vi "Legal Position Check.vi"(7 "Parameters for Legal Movements":T1, 8 "error in (no error)":errorcluster, 10 "Scope Position":refnum<vi>, 11 "Tip Coordinates":refnum<vi>) -> (0 "error out":errorcluster, 2 "Crash":bool)   [LabVIEW 2012, in "Sciscan Scope Daemon.lvlib"]
uses:
  Sciscan Scope Daemon.lvlib
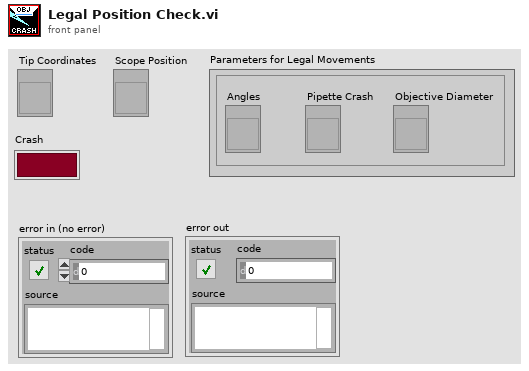
[diagram p1: front panel]
types:
  T1 = cluster{"Angles":refnum<vi>, "Objective Diameter":refnum<vi>, "Pipette Crash":refnum<vi>}
  T2 = cluster{"X [um]":dbl, "Y [um]":dbl, "Z [um]":dbl}
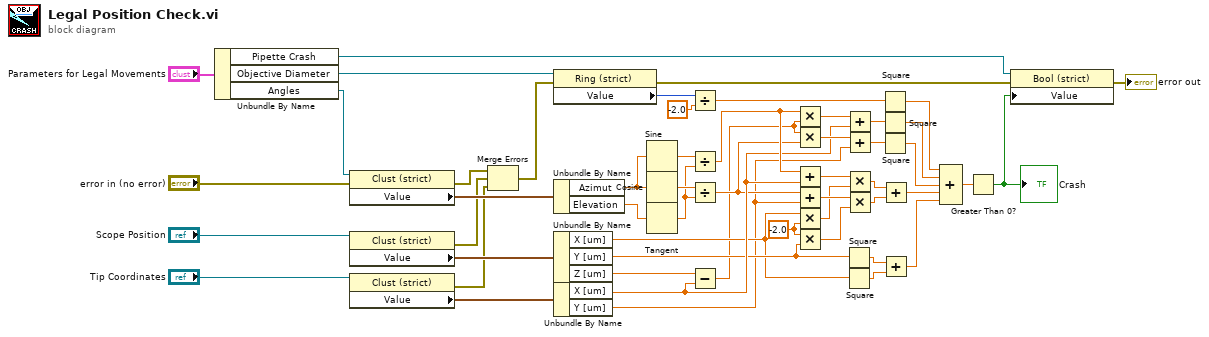
[diagram p0: block diagram]
diagram:
  w34 = -2.0 ("x")
  n1 = Unbundle By Name("Parameters for Legal Movements") -> ("Pipette Crash"=w3:refnum<vi>, "Objective Diameter"=w2:refnum<vi>, "Angles"=w1:refnum<vi>)
  n2 = property on="Property Node" class="Clust (strict)"(reference=w1, error in="error in (no error)") -> (error out=w8:errorcluster, "Value"=w17:cluster{"Azimut":dbl, "Elevation":dbl})  [unwired: 1 out]
  n3 = property on="Property Node" class="Clust (strict)"(reference="Scope Position") -> (error out=w9:errorcluster, "Value"=w15:T2)  [unwired: 1 in, 1 out]
  n4 = property on="Property Node" class="Clust (strict)"(reference="Tip Coordinates") -> (error out=w10:errorcluster, "Value"=w13:T2)  [unwired: 1 in, 1 out]
  n5 = Merge Errors(w8, w9, w10) -> (w7:errorcluster)
  n6 = property on="Property Node" class="Ring (strict)"(reference=w2, error in=w7) -> (error out=w11:errorcluster, "Value"=w12:i16)  [unwired: 1 out]
  n7 = Unbundle By Name(w17) -> ("Azimut"=w52:dbl, "Elevation"=w51:dbl)
  n8 = Unbundle By Name(w15) -> ("X [um]"=w35:dbl, "Y [um]"=w36:dbl, "Z [um]"=w47:dbl)
  n9 = Unbundle By Name(w13) -> ("X [um]"=w41:dbl, "Y [um]"=w27:dbl)
  n10 = Sine(x=w52) -> (sin(x)=w50:dbl)
  n11 = Cosine(x=w52) -> (cos(x)=w49:dbl)
  n12 = Tangent(1:w51) -> (0:w48:dbl)
  n13 = Divide(x=w12, y=-2.0) -> (x/y=w25:dbl)
  n14 = Divide(x=w50, y=w48) -> (x/y=w42:dbl)
  n15 = Divide(x=w49, y=w48) -> (x/y=w33:dbl)
  n16 = Subtract(x=w47, y=w41) -> (x-y=w32:dbl)
  n17 = Multiply(x=w42, y=w32) -> (x*y=w46:dbl)
  n18 = Multiply(x=w32, y=w33) -> (x*y=w45:dbl)
  n19 = Add(x=w42, y=w41) -> (x+y=w40:dbl)
  n20 = Add(x=w33, y=w27) -> (x+y=w39:dbl)
  n21 = Multiply(x=w35, y=w34) -> (x*y=w38:dbl)
  n22 = Multiply(x=w34, y=w36) -> (x*y=w37:dbl)
  n23 = Square(x=w36) -> (x^2=w29:dbl)
  n24 = Square(x=w35) -> (x^2=w28:dbl)
  n25 = Add(x=w46, y=w41) -> (x+y=w44:dbl)
  n26 = Add(x=w45, y=w27) -> (x+y=w43:dbl)
  n27 = Multiply(x=w40, y=w38) -> (x*y=w31:dbl)
  n28 = Multiply(x=w39, y=w37) -> (x*y=w30:dbl)
  n29 = Square(x=w25) -> (x^2=w24:dbl)
  n30 = Square(x=w44) -> (x^2=w23:dbl)
  n31 = Square(x=w43) -> (x^2=w22:dbl)
  n32 = Add(x=w31, y=w30) -> (x+y=w21:dbl)
  n33 = Add(x=w29, y=w28) -> (x+y=w20:dbl)
  n34 = Compound Arithmetic op=ADD(w24, w23, w22, w21, w20) -> (w19:dbl)
  n35 = Greater Than 0?(x=w19) -> (x > 0?=w18:bool)
  "Crash" <- w18
  n36 = property on="Property Node" class="Bool (strict)"(reference=w3, error in=w11, "Value"=w18) -> (error out=→"error out":errorcluster)  [unwired: 1 out]
